vi "tsfifo_enable_receive_fifo.vi"(8 "error in (no error)":errorcluster, 11 "Path":path) -> (0 "error out":errorcluster, 3 "Path output":path)   [LabVIEW 2014]
doc: "Function Introduction :\nEnable internal cache reception mode of the device\nCall location :\nIf an application wants to read data by accessing the cache, it should execute\nThis function must be executed before tsFifo-receive_can/canfd/lin_cessage_st\nNumber.\ninput parameter :\nnothing\nReturn value :\nnothing"
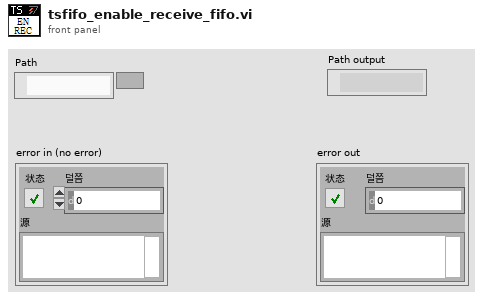
[diagram p1: front panel]
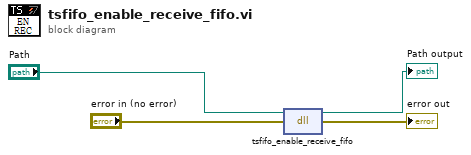
[diagram p0: block diagram]
diagram:
  n1 = dll-call lib="D:/Program Files (x86)/TOSUN/TSMaster/Data/SDK/lib/x86/TSMaster.dll" fn="tsfifo_enable_receive_fifo"(path in="Path", error in="error in (no error)") -> (path out=→"Path output":path, error out=→"error out":errorcluster)  [unwired: 2 in]
